vi "Save Data.vi"(8 "error in (no error)":errorcluster caption="错误输入（无错误）", 11 "Data":waveform(dbl)[](array[waveform]) caption="数据") -> (0 "error out":errorcluster caption="错误输出")   [LabVIEW 2013]
doc: "将数据保存至磁盘。"
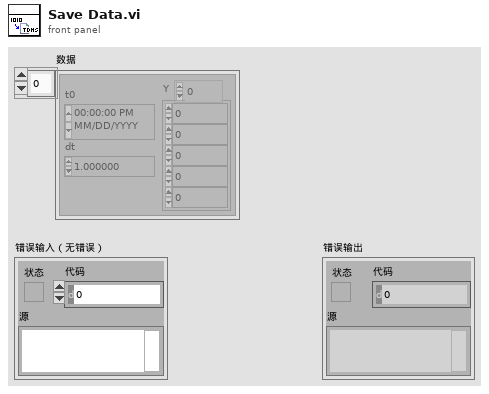
[diagram p1: front panel]
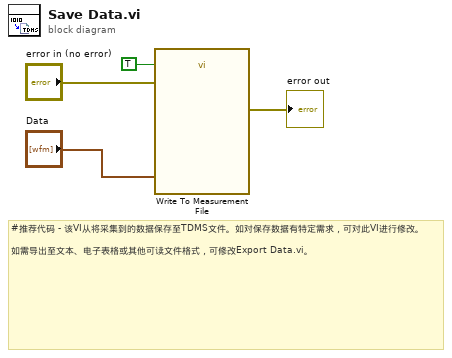
[diagram p0: block diagram]
diagram:
  # "#推荐代码 - 该VI从将采集到的数据保存至TDMS文件。如对保存数据有特定需求，可对此VI进行修改。\n\n如需导出至文本、电子表格或其他可读文件格式，可修改Export Data.vi。"
  n1 = call "Write To Measurement File"("Signals"="Data", "Reset"=TRUE, "error in (no error)"="error in (no error)") -> ("error out"=→"error out":errorcluster)  [unwired: 14 in, 2 out]
